vi "Add Virtual Instruments.vi"(6 "<JSON CFG>":string, 8 "error in":errorcluster, 11 "ICRIO MSS Test Actor in":refnum<class "ICRIO MSS Test Actor.lvclass">) -> (0 "error out":errorcluster, 3 "ICRIO MSS Test Actor out":refnum<class "ICRIO MSS Test Actor.lvclass">)   [LabVIEW 2023]
uses:
  ICRIO MSS Test Actor.lvclass
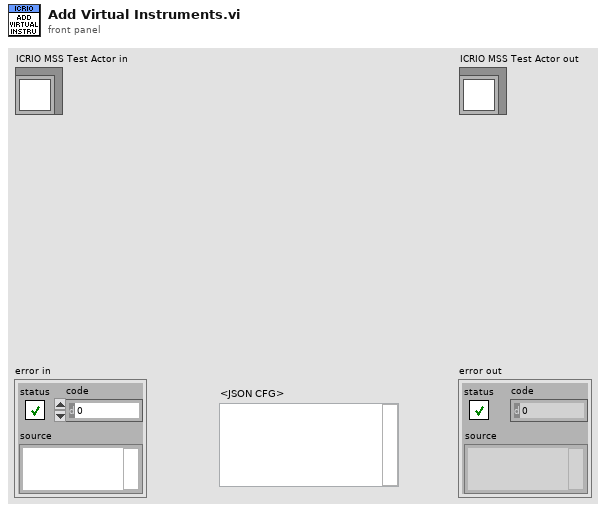
[diagram p1: front panel]
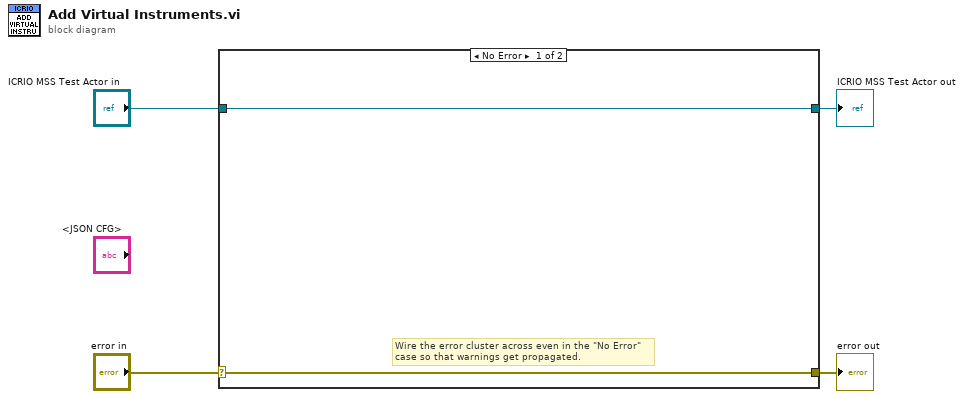
[diagram p0: block diagram]
diagram:
  n1 = case shown="No Error" "error in" {
    selector: "error in" -> [w5 w8]
    tunnel: [w5 w8] -> w3
    tunnel: [w6 w7] -> w1
    tunnel: "ICRIO MSS Test Actor in" -> [w6 w7]
    frame No Error {
      # "Wire the error cluster across even in the \"No Error\"\ncase so that warnings get propagated."
    }
    frame Error {
    }
  }
  "error out" <- w3
  "ICRIO MSS Test Actor out" <- w1
